vi "LVClasse_Phase Resize Data.vi"(0 "Phase in":refnum<class "Phase.lvclass">, 5 "Factor":u8, 7 "Resized Phase in":refnum<class "Phase.lvclass">, 9 "Erode":bool, 11 "error in (no error)":errorcluster) -> (4 "Phase out":refnum<class "Phase.lvclass">, 8 "Resized Phase out":refnum<class "Phase.lvclass">, 15 "error out":errorcluster)   [LabVIEW 2020, in "Phase.lvclass"]
doc: "Phase values buffer and pupil setter.\n\n--------------------------------------------------------------------------------\n\n<B>PhaseIn </B> : Phase object.\n<B>PhaseOut </B> : Phase object.\n<B>buffer </B> : Phase values buffer.\n<B>Pupil </B> : pupil object.\n<B>ErrorIn </B> : Error\n<B>ErrorOut </B> : Error\n\n--------------------------------------------------------------------------------"
uses:
  Phase.lvclass
  Phase.lvclass/Phase.ctl
  LVClasse_Phase Read SurfaceFloatWithPupil.vi
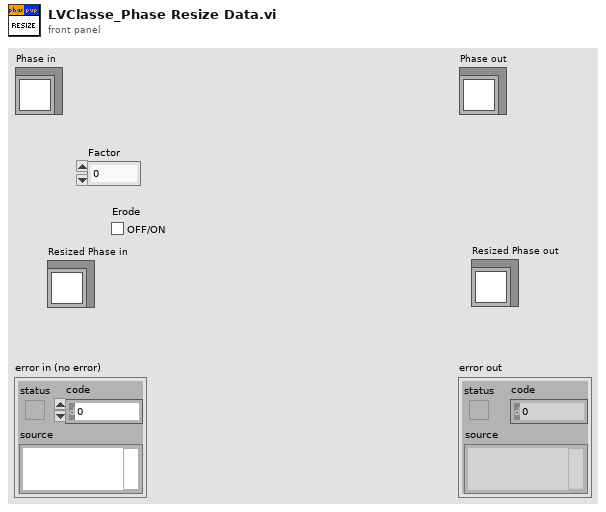
[diagram p1: front panel]
types:
  T1 = typedef "ClassID.ctl" = i64
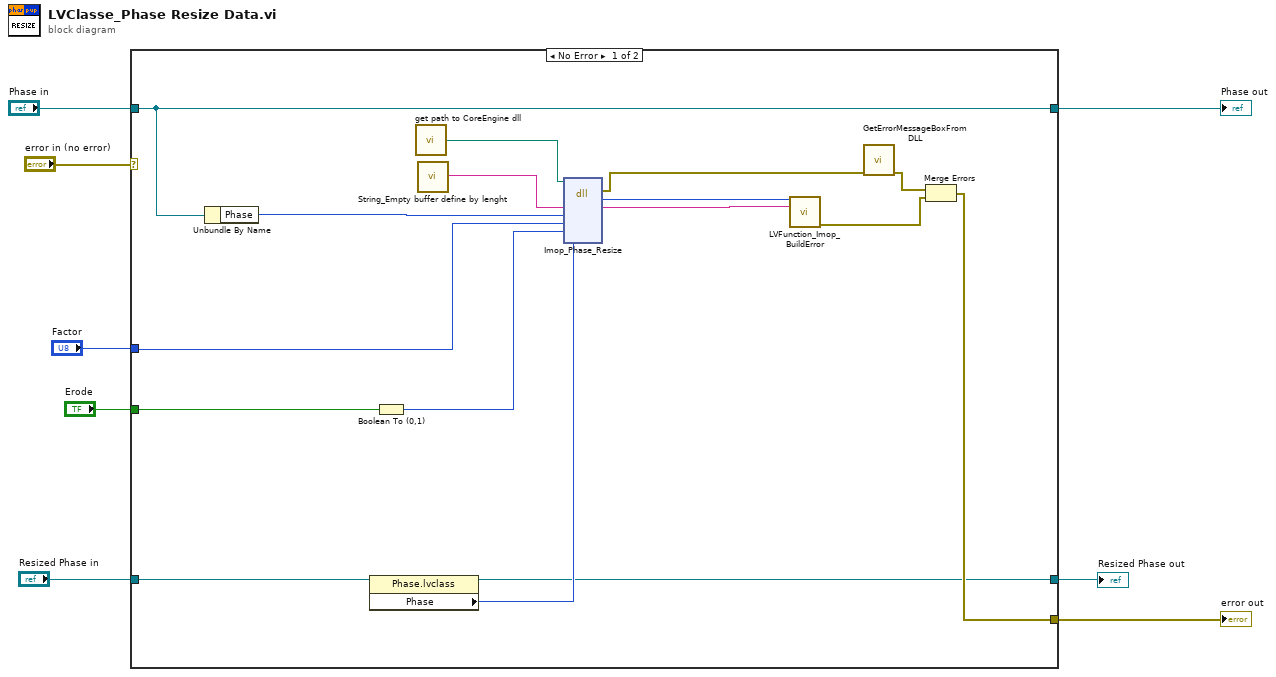
[diagram p0: block diagram]
diagram:
  n1 = case shown="No Error" "error in (no error)" {
    selector: "error in (no error)" -> [_ w27]
    tunnel: [w13 w27] -> w8
    tunnel: [w19 w26] -> w7
    tunnel: "Phase in" -> [w19 w26]
    tunnel: "Resized Phase in" -> [w17 w25]
    tunnel: "Factor" -> [w11 _]
    tunnel: [w12 w25] -> w4
    tunnel: "Erode" -> [w10 _]
    frame No Error {
      n2 = Unbundle By Name(w19) -> ("Phase"=w18:T1)
      n3 = property class="Phase.lvclass"(reference=w17) -> (reference out=w12:refnum<class "Phase.lvclass">, "Phase"=w16:T1)  [unwired: 1 in, 1 out]
      n4 = Boolean To (0,1)(Boolean=w10) -> (0, 1=w9:i16)
      n5 = call "get path to CoreEngine dll.vi"() -> ("path to wavekit library"=w21:path)  [unwired: 14 in, 1 out]
      n6 = call "String_Empty buffer define by lenght.vi"() -> ("Empty buffer"=w22:string)  [unwired: 1 in]
      n7 = dll-call lib="D:/2_trunk/Soft_haso/ImOpCoreEngine4_LV2011/DLLs/ImopEngine4_vc100.dll" fn="Imop_Phase_Resize"(path in=w21, "message"=w22, "phase"=w18, "Factor"=w11, "Erode"=w9, "resized_phase"=w16) -> (error out=w20:errorcluster, "return type"=w24:i32, "message"=w23:string)  [unwired: 6 in, 1 out]
      n8 = call "LVFunction_Imop_BuildError.vi"("code"=w24, "String to Prepend to source (\"\")"=w23) -> ("error out"=w14:errorcluster)  [unwired: 13 in]
      n9 = call "GetErrorMessageBoxFromDLL.vi"("error IN"=w20) -> ("error OUT"=w15:errorcluster)  [unwired: 10 in]
      n10 = Merge Errors(w15, w14) -> (w13:errorcluster)
    }
    frame Error {
    }
  }
  "error out" <- w8
  "Phase out" <- w7
  "Resized Phase out" <- w4
